vi "Capitalize.vi"(1 "Element":string) -> (0 "New Element":string)   [LabVIEW 2020, in "Examples.lvlib"]
doc: "An example element processor for Map.vi that capitalizes the first character of the element."
uses:
  Examples.lvlib
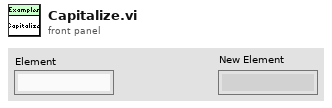
[diagram p1: front panel]
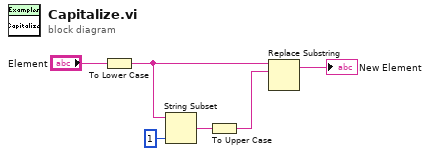
[diagram p0: block diagram]
diagram:
  n1 = To Lower Case(string="Element") -> (all lower case string=w5:string)
  n2 = String Subset(string=w5, length (rest)=1 ("length (rest)")) -> (substring=w2:string)  [unwired: 1 in]
  n3 = To Upper Case(1:w2) -> (0:w1:string)
  n4 = Replace Substring(4:w1, 5:w5) -> (1:→"New Element":string)  [unwired: 2 in, 1 out]
